vi "IsDone.vi"(0 "object in":refnum<class "BFSTreeIterator.lvclass">, 5 "Error In":errorcluster) -> (14 "object out":refnum<class "BFSTreeIterator.lvclass">, 16 "IsDone":bool, 19 "Error Out":errorcluster)   [LabVIEW 2024, in "BFSTreeIterator.lvclass"]
doc: "Return a boolean value that indicates whether traversing is done and we are at the end of the collection."
uses:
  BFSTreeIterator.lvclass
  BFSTreeIterator.lvclass/BFSTreeIterator.ctl
panel:
  # "Connector Pane"
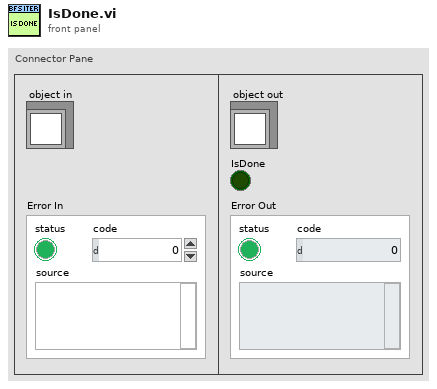
[diagram p1: front panel]
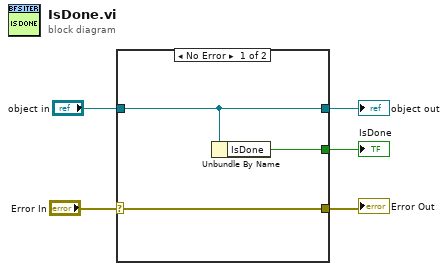
[diagram p0: block diagram]
diagram:
  n1 = case shown="No Error" "Error In" {
    selector: "Error In" -> [w8 w10]
    tunnel: [w8 w10] -> w4
    tunnel: [w7 w9] -> w2
    tunnel: "object in" -> [w7 w9]
    tunnel: [w6 _] -> w1
    frame No Error {
      n2 = Unbundle By Name(w7) -> ("IsDone"=w6:bool)
    }
    frame Error {
    }
  }
  "Error Out" <- w4
  "object out" <- w2
  "IsDone" <- w1
